vi "Enable Mute.vi"(7 "Address":u16, 8 "Error In":errorcluster, 9 "Mute (T)":bool, 10 "Detector":u8, 11 "VISA Resource in":refnum<visa-resource-name>) -> (0 "Error Out":errorcluster, 3 "VISA Resource out":refnum<visa-resource-name>)   [LabVIEW 2014, in "KIT QV.lvlib"]
doc: "Activate or deactivate time unlimited muting of selected detector."
uses:
  KIT QV.lvlib
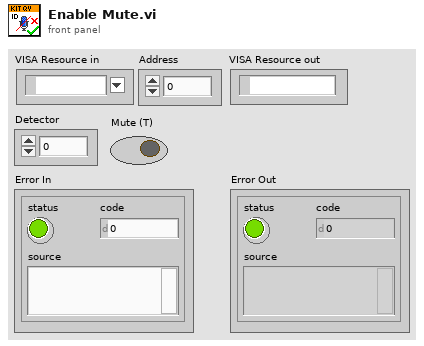
[diagram p1: front panel]
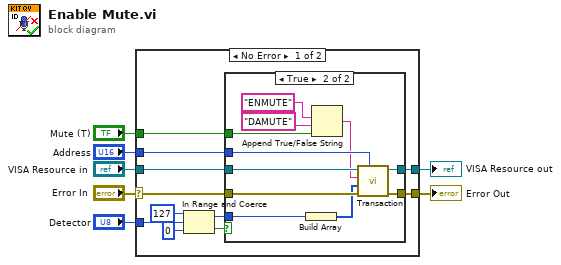
[diagram p0: block diagram]
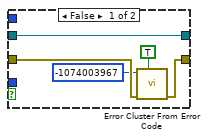
[diagram p2: hidden frame]
diagram:
  n1 = case shown="No Error" "Error In" {
    selector: "Error In" -> [w17 w35]
    tunnel: [w15 w36] -> w7
    tunnel: [w14 w35] -> w6
    tunnel: "VISA Resource in" -> [w18 w36]
    tunnel: "Address" -> [w16 _]
    tunnel: "Detector" -> [w13 _]
    tunnel: "Mute (T)" -> [w8 _]
    frame No Error {
      n2 = In Range and Coerce(upper limit=u8 127, x=w13, lower limit=u8 0) -> (coerced(x)=w10:u8, In Range?=w9:bool)
      n3 = case shown="True" w9 {
        tunnel: w18 -> [w23 w34]
        tunnel: w17 -> [w22 w33]
        tunnel: w16 -> [_ w32]
        tunnel: [w23 w31] -> w15
        tunnel: [w21 w30] -> w14
        tunnel: w10 -> [_ w29]
        tunnel: w8 -> [_ w27]
        frame False {
          n4 = call <vilib>:"Error Cluster From Error Code.vi"("show call chain? (False)"=TRUE, "error in (no error)"=w22, "error code (0)"=-1074003967) -> ("error out"=w21:errorcluster)  [unwired: 6 in]
        }
        frame True {
          n5 = Build Array(w29) -> (w28:u8[])
          n6 = Append True/False String(1:w27, 2:"DAMUTE" ("Reset Command"), 3:"ENMUTE" ("Reset Command")) -> (0:w26:string)  [unwired: 1 in]
          n7 = call "Transaction.vi"("Address"=w32, "error in (no error)"=w33, "Parameter in"=w28, "Command"=w26, "VISA Resource in"=w34) -> ("error out"=w30:errorcluster, "VISA Resource out"=w31:refnum<visa-resource-name>)  [unwired: 4 in, 1 out]
        }
      }
    }
    frame Error {
    }
  }
  "Error Out" <- w6
  "VISA Resource out" <- w7
